vi "FileDES_Decrypt.vi"(9 "加密后的文件":path, 10 "秘钥":path, 11 "被加密的文件":path) -> (3 "返回值":i32)   [LabVIEW 2011]
uses:
  Data/DES.dll
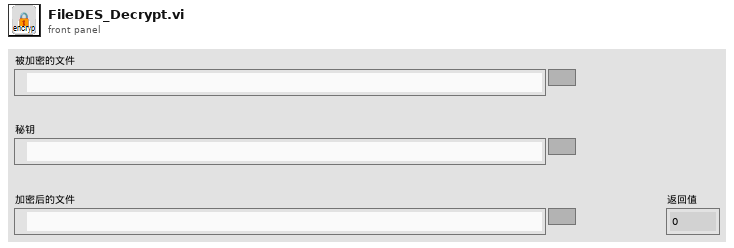
[diagram p1: front panel]
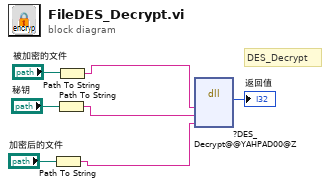
[diagram p0: block diagram]
diagram:
  # "DES_Decrypt"
  n1 = Path To String(path="加密后的文件") -> (string=w4:string)
  n2 = Path To String(path="秘钥") -> (string=w5:string)
  n3 = Path To String(path="被加密的文件") -> (string=w6:string)
  n4 = dll-call lib="PTH1Vabs D高频房软件-2. HPTS_VNA_Rev2.7.1.3-0327最新源码备份DataDES.dll" fn="?DES_Decrypt@@YAHPAD00@Z"("cipherFile"=w6, "keyStr"=w5, "plainFile"=w4) -> ("返回类型"=→"返回值":i32)  [unwired: 6 in, 2 out]
